vi "HP amount.vi"() -> ()   [LabVIEW 2025]
panel:
  out "HP amount":u32
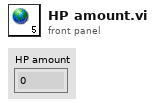
[diagram p1: front panel]
diagram:
